vi "QX_Get Signals.vi"(7 "QX Dev.QX DevInfo[]":T2[](array[typedef]), 8 "Error in":errorcluster, 10 "FirstSignalsOnly":bool=TRUE, 11 "ModRef[]":refnum<k24>[](array[refnum])) -> (0 "Error out":errorcluster, 2 "QXModuInfo":T2[](array[typedef]), 5 "DevRef[]":T1(array[cluster]))   [LabVIEW 2016]
doc: "Delivers (all) signals of the given devices.\n\nDevices: Devices from which to deliver the signals\nFirstSignalsOnly: Set to true (default) if you only want the get the respective first signals of each channel (QuantumX devices return 2 signals per channel if FirstSignalsOnly is set to false).\n\nDevicesAndSignals: Cluster consisting of an array of devices and an array of all signals of the given devices"
uses:
  QX Module Info.ctl
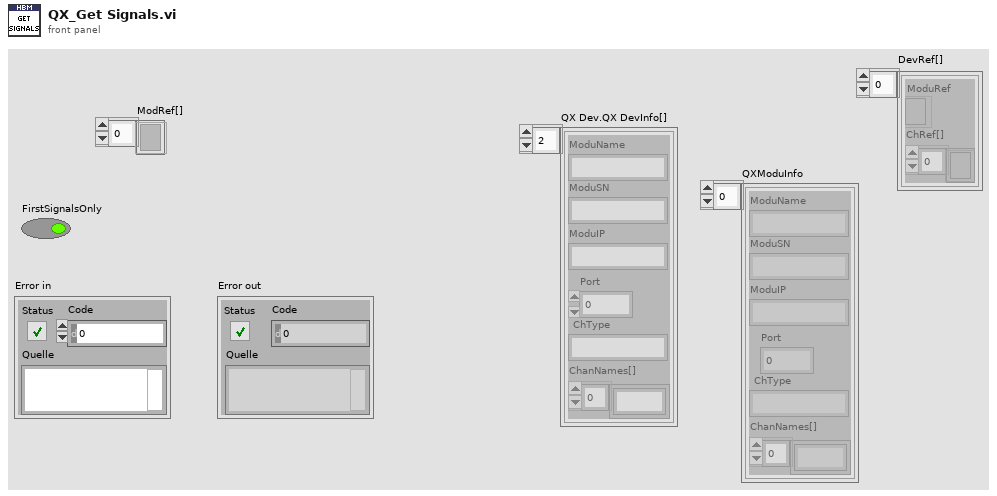
[diagram p1: front panel]
types:
  T1 = cluster{"ModuRef":refnum<k24>, "ChRef[]":refnum<k24>[]}[]
  T2 = typedef "QX Module Info.ctl" = cluster{"ModuName":string, "ModuSN":string, "ModuIP":string, "Port":i32, "ChType":string, "ChanNames[]":string[]}
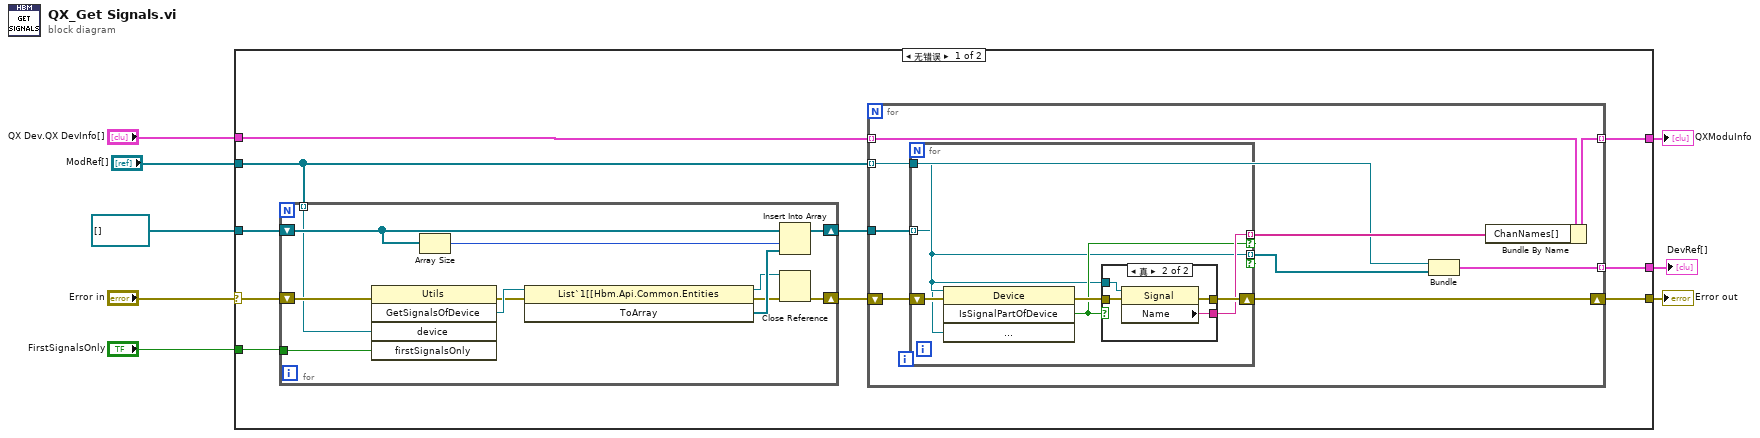
[diagram p0: block diagram]
diagram:
  n1 = case shown="无错误" "Error in" {
    selector: "Error in" -> [w17 w51]
    tunnel: [w16 w51] -> w8
    tunnel: "FirstSignalsOnly" -> [w15 _]
    tunnel: [w14 _] -> w5
    tunnel: "QX Dev.QX DevInfo[]" -> [w11 _]
    tunnel: refnum<k24>[] [] -> [w12 _]
    tunnel: "ModRef[]" -> [w10 _]
    tunnel: [w9 _] -> w1
    frame No Error {
      n2 = for {
        shift-right: [w50] -> w13
        shift-left: w12 -> [w49]
        shift-right: [w41] -> w16
        shift-left: w17 -> [w45]
        tunnel: w15 -> [w44]
        tunnel: w10 -> [w39] mode=indexing
        n3 = invoke on="Methodenknoten" class="Utils" method="GetSignalsOfDevice"(error in=w45, "device"=w39, "firstSignalsOnly"=w44) -> (error out=w46:errorcluster, "GetSignalsOfDevice"=w47:refnum<k24>)  [unwired: 2 in, 3 out]
        n4 = Array Size(array=w49) -> (size(s)=w48:i32)
        n5 = invoke on="Methodenknoten" class="List`1[[Hbm.Api.Common.Entities" method="ToArray"(reference=w47, error in=w46) -> (reference out=w40:refnum<k24>, error out=w42:errorcluster, "ToArray"=w43:refnum<k24>[])  [unwired: 1 in]
        n6 = Insert Into Array(array=w49, index=w48, new element=w43) -> (w50:refnum<k24>[])
        n7 = Close Reference(reference=w40, error in (no error)=w42) -> (error out=w41:errorcluster)
      }
      n8 = for {
        tunnel: w13 -> [w26]
        shift-right: [w25] -> _
        shift-left: _ -> [w24]
        tunnel: [w22] -> w14 mode=indexing
        tunnel: w11 -> [w21] mode=indexing
        tunnel: w10 -> [w20] mode=indexing
        tunnel: [w18] -> w9 mode=indexing
        n9 = for {
          tunnel: w20 -> [w33]
          tunnel: w26 -> [w27] mode=indexing
          shift-right: [w30] -> w25
          shift-left: w24 -> [w32]
          tunnel: [w29] -> w23 mode=indexing if=w28
          tunnel: [w27] -> w19 mode=indexing if=w28
          n10 = invoke on="Methodenknoten" class="Device" method="IsSignalPartOfDevice"(reference=w33, error in=w32, "signalToCheck"=w27) -> (error out=w31:errorcluster, "IsSignalPartOfDevice"=w28:bool)  [unwired: 1 in, 2 out]
          n11 = case shown="真" w28 {
            tunnel: w31 -> [w34 w37]
            tunnel: w27 -> [_ w38]
            tunnel: [w34 w36] -> w30
            tunnel: [_ w35] -> w29
            frame False {
            }
            frame True {
              n12 = property on="Eigenschaftsknoten" class="Signal"(reference=w38, error in=w37) -> (error out=w36:errorcluster, "Name"=w35:string)  [unwired: 1 out]
            }
          }
        }
        n13 = Bundle(w20, w19) -> (w18:cluster{refnum<k24>, refnum<k24>[]})  [unwired: 1 in]
        n14 = Bundle By Name(cluster=w21, "ChanNames[]"=w23) -> (w22:T2)
      }
    }
    frame Error {
    }
  }
  "Error out" <- w8
  "QXModuInfo" <- w5
  "DevRef[]" <- w1
